vi "WPI_UltrasonicRefNum Registry Get.vi"   [LabVIEW 2017]
doc: "Gets the reference you specify. You first must set the reference with the RefNum Registry Set VI."
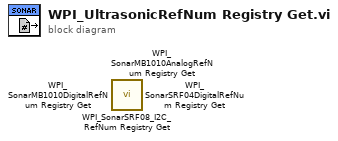
[diagram p0: block diagram]
diagram:
  n1 = call <vilib>:"WPI_SonarSRF08_I2C_RefNum Registry Get.vi"() -> ()  [unwired: 10 in, 2 out]
  n2 = call <vilib>:"WPI_SonarMB1010AnalogRefNum Registry Get.vi"() -> ()  [unwired: 10 in, 2 out]
  n3 = call <vilib>:"WPI_SonarMB1010DigitalRefNum Registry Get.vi"() -> ()  [unwired: 10 in, 2 out]
  n4 = call <vilib>:"WPI_SonarSRF04DigitalRefNum Registry Get.vi"() -> ()  [unwired: 10 in, 2 out]
